vi "CameraDisplay.vi"(11 "Image Display 2":T1) -> (0 "error constant":errorcluster)   [LabVIEW 2023]
uses:
  <vilib>/vision/Image Controls.llb/IMAQ Image.ctl
panel:
  out "Image Display":T1(plugin-control)
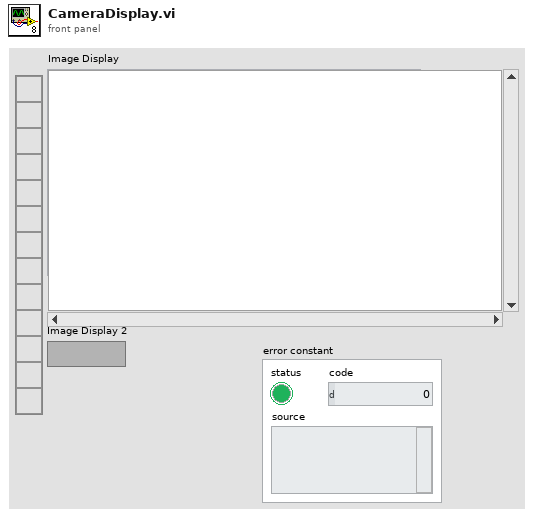
[diagram p1: front panel]
types:
  T1 = typedef "IMAQ Image.ctl" = refnum<image>
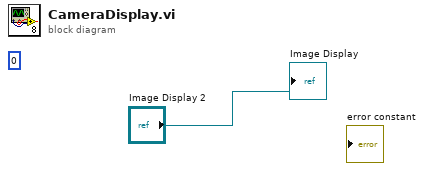
[diagram p0: block diagram]
diagram:
  (unwired) 0
  "Image Display" <- "Image Display 2"
